vi "Flatten To JSON String.vi"(4 "Enums As String (F)":bool, 5 "Numeric Extensions (F)":bool, 6 "Timestamp Options":T1={"Convert Timestamps"=TRUE, "UTC"=TRUE}, 7 "Multiline (T)":bool=TRUE, 8 "error in (no error)":errorcluster, 11 "Variant":variant) -> (0 "error out":errorcluster, 3 "JSON String":string)   [LabVIEW 2020, in "JKI JSON Object Serialization.lvlib"]
doc: "Converts <b>Variant</b> to <b>JSON String</b>. Accepts LabVIEW class objects as input. If <b>Multiline</b> is false returns a single-line JSON string, otherwise returns a pretty-printed multi-line string. If <b>Numeric Extensions</b> is true, converts +-Inf and NaN to symbolic values compatible with many JSON libraries but not part of JSON standard. If <b>Convert Timestamps</b> is true in <b>Timestamp Options</b> converts LabVIEW timestamps to ISO timestamp strings. If <b>UTC</b>is true, uses universal time instead of local time. \n\nGCraftsman JSON Object Serialization Toolkit\nwww.GCraftsman.com\nCopyright (c) 2017, GCraftsman"
uses:
  JKI JSON Object Serialization.lvlib
  <vilib>/addons/_JKI.lib/Serialization/JSON/Library/Timestamp Options.ctl
  Serializer/Serializer.lvclass
  <vilib>/addons/_JKI.lib/Serialization/JSON/JKI JSON Serialization.lvlib
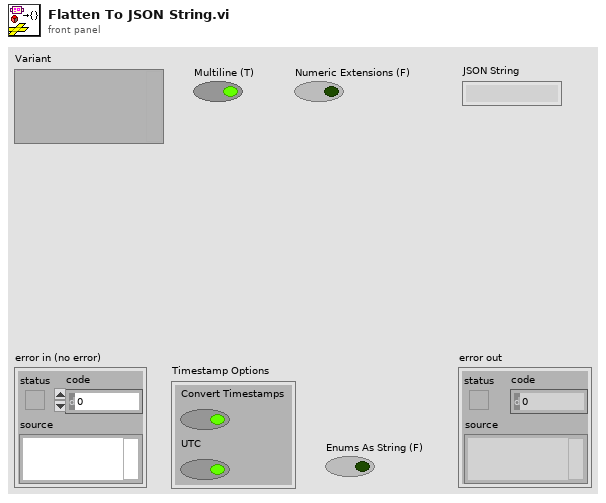
[diagram p1: front panel]
types:
  T1 = typedef "JKI JSON Serialization.lvlib/Timestamp Options.ctl" = cluster{"Convert Timestamps":bool, "UTC":bool}
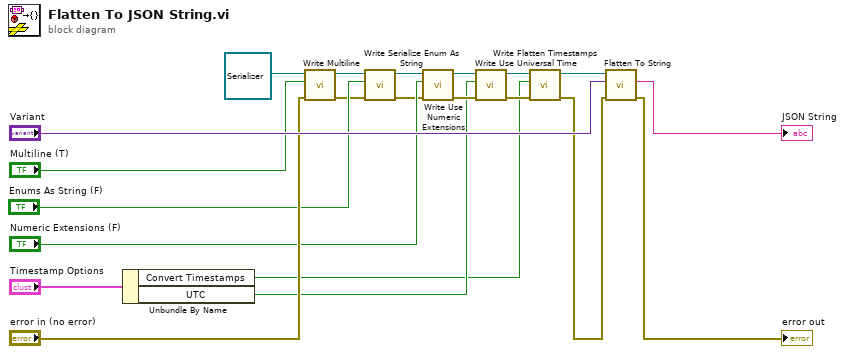
[diagram p0: block diagram]
diagram:
  n1 = Unbundle By Name("Timestamp Options") -> ("Convert Timestamps"=w7:bool, "UTC"=w8:bool)
  n2 = call-dynamic "Write Multiline.vi"("error in (no error)"="error in (no error)", "Multiline"="Multiline (T)", "JSON Serializer in"=refnum<class "Serializer.lvclass"> refnum ("JSON Object Serializer.lvclass")) -> ("error out"=w4:errorcluster, "JSON Serializer out"=w6:refnum<class "Serializer.lvclass">)  [unwired: 7 in]
  n3 = call-dynamic "Write Serialize Enum As String.vi"("error in (no error)"=w4, "Enums As String"="Enums As String (F)", "JSON Serializer in"=w6) -> ("error out"=w3:errorcluster, "JSON Serializer out"=w2:refnum<class "Serializer.lvclass">)  [unwired: 7 in]
  n4 = call-dynamic "Write Use Numeric Extensions.vi"("error in (no error)"=w3, "Numeric Extensions"="Numeric Extensions (F)", "JSON Serializer in"=w2) -> ("error out"=w16:errorcluster, "JSON Serializer out"=w17:refnum<class "Serializer.lvclass">)  [unwired: 7 in]
  n5 = call-dynamic "Write Use Universal Time.vi"("error in (no error)"=w16, "Universal Time"=w8, "JSON Serializer in"=w17) -> ("error out"=w15:errorcluster, "JSON Serializer out"=w18:refnum<class "Serializer.lvclass">)  [unwired: 7 in]
  n6 = call-dynamic "Write Flatten Timestamps.vi"("error in (no error)"=w15, "Convert Timestamps"=w7, "JSON Serializer in"=w18) -> ("error out"=w13:errorcluster, "JSON Serializer out"=w12:refnum<class "Serializer.lvclass">)  [unwired: 7 in]
  n7 = call-dynamic "Flatten To String.vi"("error in (no error)"=w13, "Variant"="Variant", "JSON Object Serializer in"=w12) -> ("error out"=→"error out":errorcluster, "String"=→"JSON String":string)  [unwired: 6 in, 1 out]
